vi "ADC config.vi"(8 "error in (no error)":errorcluster, 9 "Opciones":T1(ring), 10 "Write":string, 11 "VISA Refnum in":refnum<visa-resource-name>) -> (0 "error out":errorcluster, 3 "Read":string)   [LabVIEW 2020, in "Arduino.lvclass"]
uses:
  Arduino.lvclass
  <vilib>/Instr/_visa.llb/VISA Configure Serial Port (Instr).vi
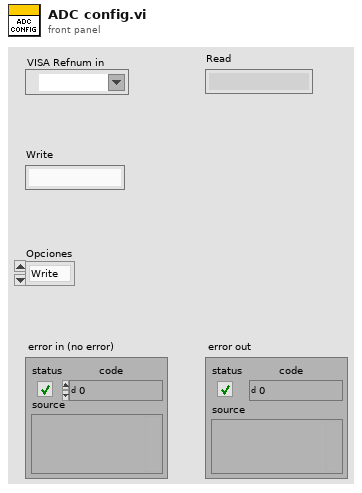
[diagram p1: front panel]
types:
  T1 = enum16{"Write", "Read", "Config", "Reset", "Close"}
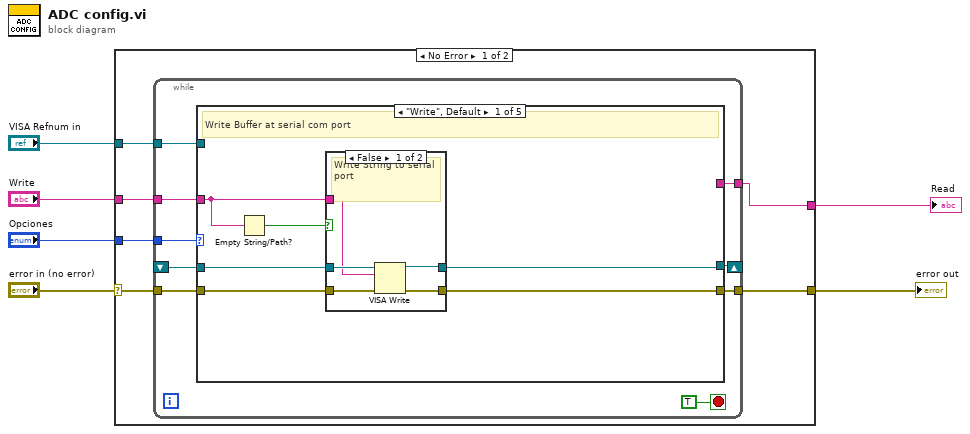
[diagram p0: block diagram]
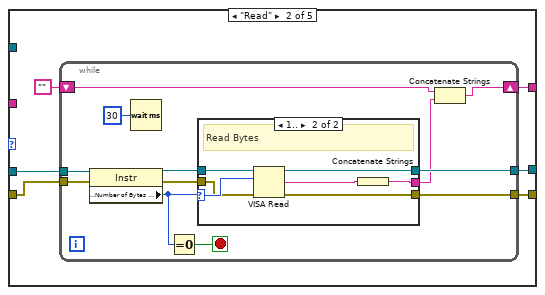
[diagram p3: hidden frame]
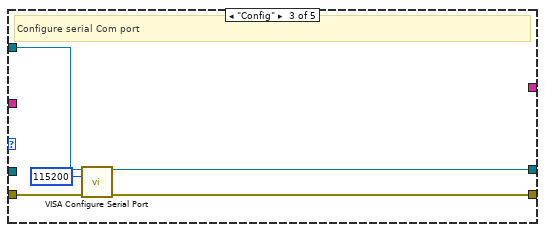
[diagram p5: hidden frame]
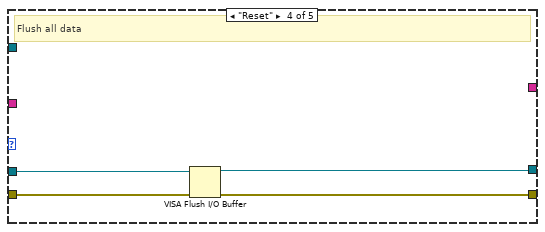
[diagram p6: hidden frame]
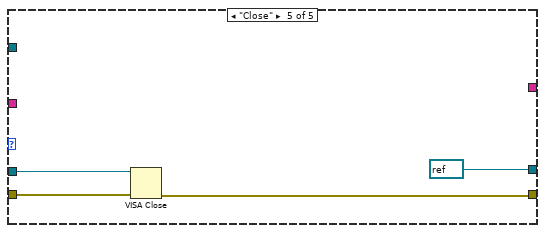
[diagram p7: hidden frame]
diagram:
  n1 = case shown="No Error" "error in (no error)" {
    selector: "error in (no error)" -> [w11 w75]
    tunnel: [w10 w75] -> w2
    tunnel: "Opciones" -> [w12 _]
    tunnel: "VISA Refnum in" -> [w9 _]
    tunnel: "Write" -> [w8 _]
    tunnel: [w7 _] -> w6
    frame No Error {
      n2 = while {
        tunnel: w12 -> [w20]
        tunnel: w11 -> [w19]
        tunnel: [w18] -> w10
        tunnel: w9 -> [w17]
        shift-right: [w16] -> _
        shift-left: _ -> [w15]
        tunnel: w8 -> [w14]
        tunnel: [w13] -> w7
        stop <- TRUE stop-if-true
        n3 = case shown="\"Write\", Default" w20 {
          tunnel: w19 -> [w27 w39 w66 w70 w74]
          tunnel: [w26 w38 w62 w69 w73] -> w18
          tunnel: w17 -> [_ _ w65 _ _]
          tunnel: [w22 w37 w64 w67 refnum<visa-resource-name> refnum ("VISA resource name out")] -> w16
          tunnel: w15 -> [w25 w40 _ w68 w72]
          tunnel: w14 -> [w24 _ _ _ _]
          tunnel: [_ w36 _ _ _] -> w13
          frame "Write", Default {
            # "Write Buffer at serial com port"
            n4 = Empty String/Path?(string/path=w24) -> (empty?=w23:bool)
            n5 = case shown="False" w23 {
              tunnel: w27 -> [w32 w33]
              tunnel: [w31 w33] -> w26
              tunnel: w25 -> [w30 w34]
              tunnel: w24 -> [w29 _]
              tunnel: [w28 w34] -> w22
              frame False {
                # "Write String to serial port"
                n6 = VISA Write(VISA resource name=w30, write buffer=w29, error in (no error)=w32) -> (VISA resource name out=w28:refnum<visa-resource-name>, error out=w31:errorcluster)  [unwired: 1 out]
              }
              frame True {
              }
            }
          }
          frame "Read" {
            n7 = while {
              tunnel: w40 -> [w52]
              tunnel: w39 -> [w51]
              tunnel: [w48] -> w38
              tunnel: [w47] -> w37
              shift-right: [w42] -> w36
              shift-left: "" -> [w41]
              stop <- w44 stop-if-true
              n8 = property class="Instr"(reference=w52, error in=w51) -> (reference out=w50:refnum<visa-resource-name>, error out=w49:errorcluster, "Serial Settings:Number of Bytes at Serial Port"=w45:u32)
              n9 = Wait (ms)(milliseconds to wait=u32 30) -> ()  [unwired: 1 out]
              n10 = Equal To 0?(x=w45) -> (x = 0?=w44:bool)
              n11 = case shown="1.." w45 {
                selector: w45 -> [_ w60]
                tunnel: w50 -> [w54 w61]
                tunnel: w49 -> [w53 w57]
                tunnel: [w53 w59] -> w48
                tunnel: [w54 w58] -> w47
                tunnel: [_ w55] -> w43
                frame 0, Default {
                }
                frame 1.. {
                  # "Read Bytes"
                  n12 = VISA Read(VISA resource name=w61, byte count=w60, error in (no error)=w57) -> (VISA resource name out=w58:refnum<visa-resource-name>, read buffer=w56:string, error out=w59:errorcluster)  [unwired: 1 out]
                  n13 = Concatenate Strings(w56) -> (w55:string)
                }
              }
              n14 = Concatenate Strings(w41, w43) -> (w42:string)
            }
          }
          frame "Config" {
            # "Configure serial Com port"
            n15 = call-poly "VISA Configure Serial Port"("VISA resource name"=w65, "baud rate (9600)"=u32 115200, "error in (no error)"=w66) -> ("VISA resource name out"=w64:refnum<visa-resource-name>, "error out"=w62:errorcluster)  [unwired: 11 in]
          }
          frame "Reset" {
            # "Flush all data"
            n16 = VISA Flush I/O Buffer(VISA resource name=w68, error in (no error)=w70) -> (VISA resource name out=w67:refnum<visa-resource-name>, error out=w69:errorcluster)  [unwired: 1 in]
          }
          frame "Close" {
            n17 = VISA Close(VISA resource name=w72, error in (no error)=w74) -> (error out=w73:errorcluster)
          }
        }
      }
    }
    frame Error {
    }
  }
  "error out" <- w2
  "Read" <- w6
